vi "SbigAdaptWindow.vi"(2 "Window in":T1, 3 "Binning Mode":u16(ring) items=["1x1", "2x2", "3x3"]) -> (0 "Window out":T1, 1 "Window out 2":T1)   [LabVIEW 2009]
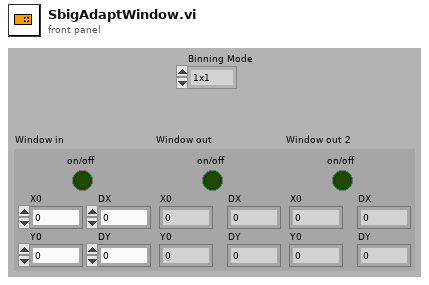
[diagram p1: front panel]
types:
  T1 = cluster{"X0":u16, "Y0":u16, "DX":u16, "DY":u16, "on/off":bool}
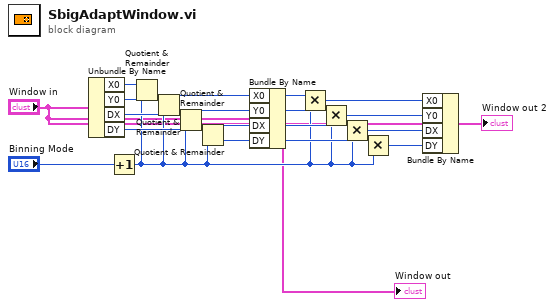
[diagram p0: block diagram]
diagram:
  n1 = Unbundle By Name("Window in") -> ("X0"=w14:u16, "Y0"=w17:u16, "DX"=w16:u16, "DY"=w15:u16)
  n2 = Increment(x="Binning Mode") -> (x+1=w9:u16)
  n3 = Quotient & Remainder(x=w14, y=w9) -> (floor(x/y)=w13:u16)  [unwired: 1 out]
  n4 = Quotient & Remainder(x=w17, y=w9) -> (floor(x/y)=w12:u16)  [unwired: 1 out]
  n5 = Quotient & Remainder(x=w16, y=w9) -> (floor(x/y)=w11:u16)  [unwired: 1 out]
  n6 = Quotient & Remainder(x=w15, y=w9) -> (floor(x/y)=w10:u16)  [unwired: 1 out]
  n7 = Bundle By Name(cluster="Window in", "X0"=w13, "Y0"=w12, "DX"=w11, "DY"=w10) -> (→"Window out":T1)
  n8 = Multiply(x=w13, y=w9) -> (x*y=w8:u16)
  n9 = Multiply(x=w12, y=w9) -> (x*y=w7:u16)
  n10 = Multiply(x=w11, y=w9) -> (x*y=w6:u16)
  n11 = Multiply(x=w10, y=w9) -> (x*y=w5:u16)
  n12 = Bundle By Name(cluster="Window in", "X0"=w8, "Y0"=w7, "DX"=w6, "DY"=w5) -> (→"Window out 2":T1)
